vi "GotoWaypoint.vi"(7 "InhibitIn":bool, 8 "CurrentSteerAngle":dbl, 9 "WhatAroundMe? Clean":cluster{"T":dbl, "Range":dbl, "Bearing":dbl}[](array[cluster]), 10 "WhereAmI? Clean":T3, 11 "MDF In":T2(array[cluster])) -> (0 "BehCom":T1(ring), 1 "MDF Out":T2(array[cluster]), 2 "ActCommand":dbl[](array[numeric]), 4 "InhibitOut":bool, 5 "Vel":dbl, 6 "SteerAngle":dbl)   [LabVIEW 2012]
doc: "This subVI contains the Forebrain Goto Waypoint behaviors. Its inputs are the outputs of thewhat and where SENSE processes, theMission efinition Filet, a suppression value from another co-brahvior and an inhibit signal to turn the behavior off. The outputs are a 90 element steering array and a suppression value to diminish the output of co-behaviors.\n\nIt is designed to work with a 90 element behavior arbiter."
uses:
  <vilib>/Analysis/1siggen.llb/Ramp Pattern by Samples.vi
  <vilib>/gmath/statdist.llb/Normal PDF.vi
  <vilib>/gmath/NI_Gmath.lvlib
  <vilib>/Analysis/NI_AALBase.lvlib
panel:
  out "loop index":i32
  in  "HowAmI? Clean":cluster{"T":dbl, "Battery":dbl, "Temp":dbl}
  # "This VI contains the go to waypoint behavior  at the Forebrain level"
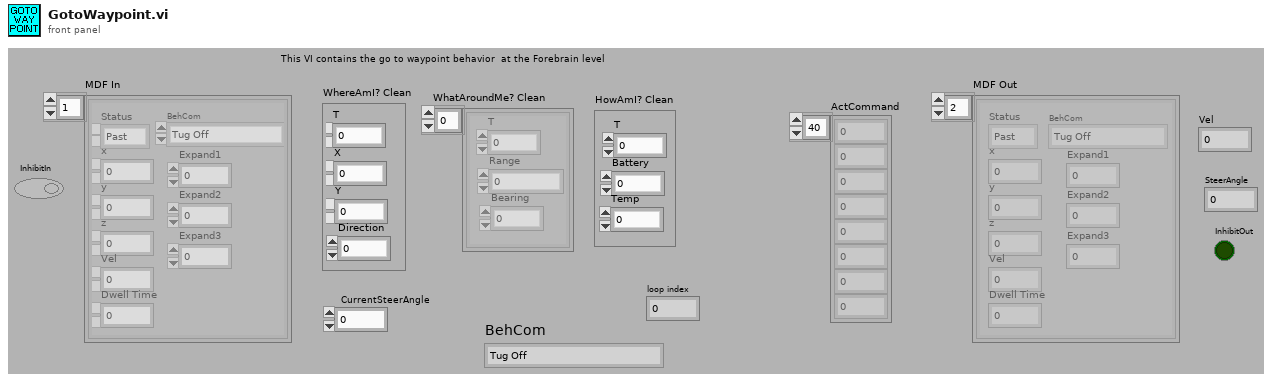
[diagram p1: front panel]
types:
  T1 = enum16{"Tug Off", "Manual Mode", "Goto WayPoint", "Back Up", "Circle", "Left Wall Follow", "Right Wall Follow", "Hunt"}
  T2 = cluster{"Status":enum16{"Past", "Current", "Future"}, "x":dbl, "y":dbl, "z":dbl, "Vel":dbl, "Dwell Time":dbl, "BehCom":enum16{"Tug Off", "Manual Mode", "Goto WayPoint", "Back Up", "Circle", "Left Wall Follow", "Right Wall Follow", "Hunt"}, "Expand1":dbl, "Expand2":dbl, "Expand3":dbl}[]
  T3 = cluster{"T":dbl, "X":dbl, "Y":dbl, "Direction":dbl}
  T4 = cluster{"Status":enum16{"Past", "Current", "Future"}, "x":dbl, "y":dbl, "z":dbl, "Vel":dbl, "Dwell Time":dbl, "BehCom":enum16{"Tug Off", "Manual Mode", "Goto WayPoint", "Back Up", "Circle", "Left Wall Follow", "Right Wall Follow", "Hunt"}, "Expand1":dbl, "Expand2":dbl, "Expand3":dbl}
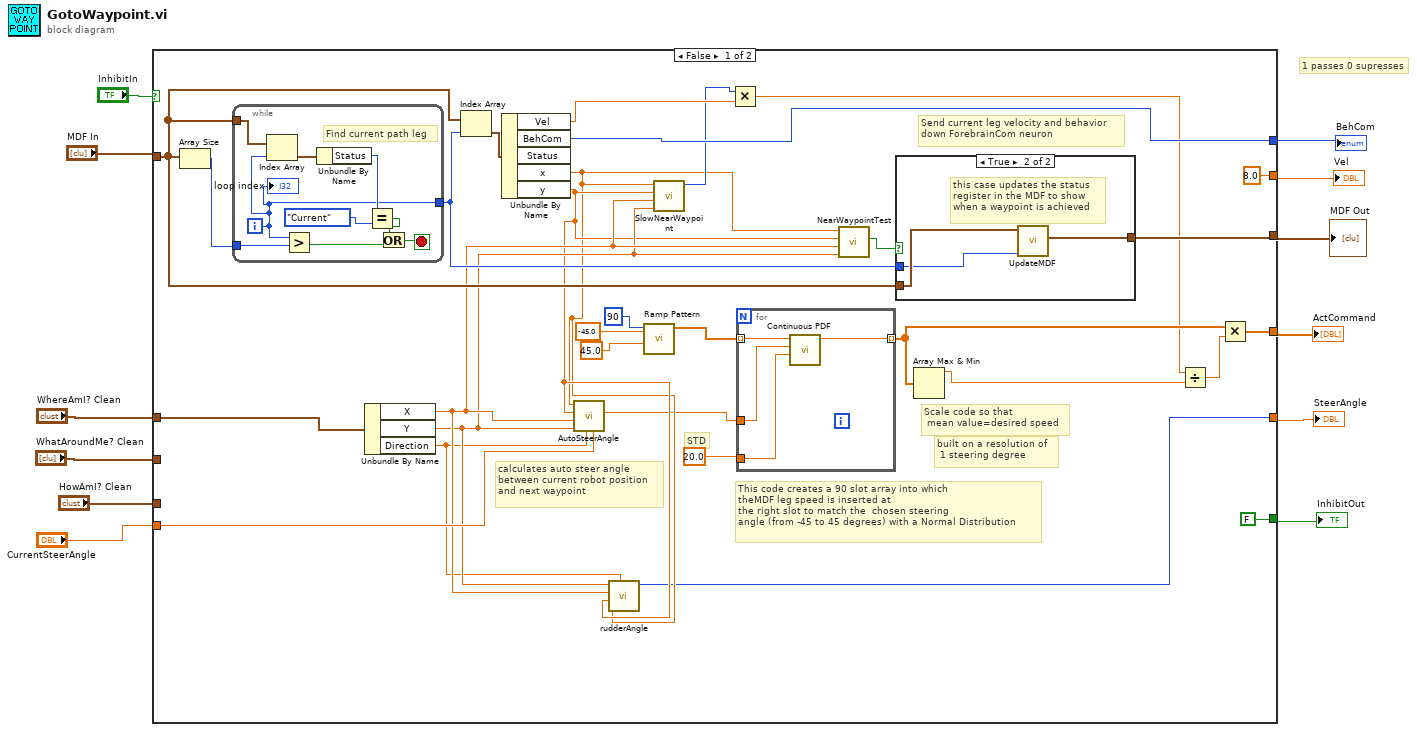
[diagram p0: block diagram]
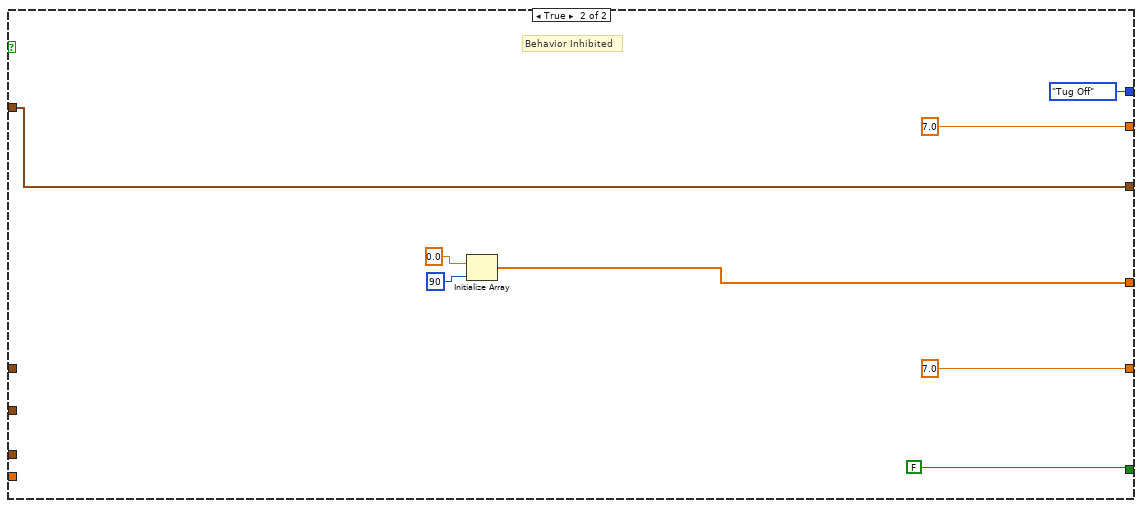
[diagram p3: hidden frame]
diagram:
  # "1 passes 0 supresses"
  n1 = case shown="False" "InhibitIn" {
    tunnel: "WhatAroundMe? Clean" -> [_ _]
    tunnel: "WhereAmI? Clean" -> [w40 _]
    tunnel: "HowAmI? Clean" -> [_ _]
    tunnel: [w30 w66] -> w7
    tunnel: [FALSE ("InhibitOut") FALSE ("InhibitOut")] -> w8
    tunnel: "MDF In" -> [w28 w63]
    tunnel: [w27 w63] -> w5
    tunnel: [8.0 ("Vel") 7.0 ("Vel")] -> w4
    tunnel: [w14 7.0 ("SteerAngle")] -> w3
    tunnel: "CurrentSteerAngle" -> [w25 _]
    tunnel: [w24 T1."Tug Off" ("BehCom")] -> w1
    frame False {
      # "Send current leg velocity and behavior\ndown ForebrainCom neuron"
      # "calculates auto steer angle\nbetween current robot position\nand next waypoint"
      # "built on a resolution of\n 1 steering degree"
      # "Scale code so that\n mean value=desired speed"
      # "STD"
      # "This code creates a 90 slot array into which\ntheMDF leg speed is inserted at\nthe right slot to match the  chosen steering\nangle (from -45 to 45 degrees) with a Normal Distribution"
      n2 = Array Size(array=w28) -> (size(s)=w41:i32)
      n3 = while {
        tunnel: w41 -> [w59]
        tunnel: w28 -> [w56]
        tunnel: [w51] -> w26
        i -> [w51]
        stop <- w58 stop-if-true
        # "Find current path leg"
        n4 = Index Array "Index Array"(array=w56, index=w51) -> (element=w53:T4)
        n5 = Greater?(x=w51, y=w59) -> (0:w57:bool)
        n6 = Unbundle By Name(w53) -> ("Status"=w54:enum16{"Past", "Current", "Future"})
        n7 = Equal?(x=w54, y=enum16{"Past", "Current", "Future"}."Current") -> (x = y?=w55:bool)
        n8 = Or(x=w55, y=w57) -> (x .or. y?=w58:bool)
        "loop index" <- w51
      }
      n9 = Unbundle By Name(w40) -> ("X"=w20:dbl, "Y"=w19:dbl, "Direction"=w18:dbl)
      n10 = Index Array "Index Array"(array=w28, index=w26) -> (element=w39:T4)
      n11 = Unbundle By Name(w39) -> ("Vel"=w23:dbl, "BehCom"=w24:T1, "x"=w16:dbl, "y"=w17:dbl)  [unwired: 1 out]
      n12 = call "AutoSteerAngle.vi"("CurrentSteerAngle"=w25, "CurrentDirection"=w18, "Ycurrent"=w19, "Xcurrent"=w20, "Ywaypoint"=w17, "Xwaypoint"=w16) -> ("NewSteerAngle"=w15:dbl)  [unwired: 5 in]
      n13 = call "rudderAngle.vi"("BoatHeading"=w18, "YGoal"=w16, "XGoal"=w17, "Yboat"=w20, "Xboat"=w19) -> ("RudderAngle"=w14:i16)  [unwired: 1 in, 2 out]
      n14 = call-poly <vilib>:"Ramp Pattern.vi"("start"=45.0, "end"=-45.0 ("end (Normal)"), "samples"=90) -> ("Ramp Pattern"=w33:dbl[])  [unwired: 7 in, 1 out]
      n15 = call "SlowNearWaypoint.vi"("Yrobot"=w19, "Xrobot"=w20, "Ywaypoint"=w17, "Xwaypoiny"=w16) -> ("SpeedDecrease"=w21:i32)  [unwired: 7 in]
      n16 = Multiply(x=w21, y=w23) -> (x*y=w22:dbl)
      n17 = for {
        tunnel: w33 -> [w50] mode=indexing
        tunnel: 20.0 ("std (Normal)") -> [w49]
        tunnel: [w48] -> w37 mode=indexing
        tunnel: w15 -> [w47]
        n18 = call-poly <vilib>:"Continuous PDF.vi"("std"=w49, "mean"=w47, "x"=w50) -> ("pdf(x)"=w48:dbl)  [unwired: 7 in, 1 out]
      }
      n19 = call "NearWaypointTest.vi"("Yrobot"=w19, "Xrobot"=w20, "Ywaypoint"=w17, "Xwaypoiny"=w16) -> ("AtWaypoint"=w29:bool)  [unwired: 7 in]
      n20 = case shown="True" w29 {
        tunnel: w28 -> [w43 w46]
        tunnel: [w43 w44] -> w27
        tunnel: w26 -> [_ w45]
        frame False {
          # "robot not near waypoint\npass MDF through unaltered"
        }
        frame True {
          # "this case updates the status\nregister in the MDF to show \nwhen a waypoint is achieved"
          n21 = call "UpdateMDF.vi"("Index"=w45, "MDF_In"=w46) -> ("MDF_Out"=w44:T2)  [unwired: 9 in]
        }
      }
      n22 = Array Max & Min(array=w37) -> (max value=w35:dbl)  [unwired: 3 out]
      n23 = Divide(x=w22, y=w35) -> (x/y=w36:dbl)
      n24 = Multiply(x=w37, y=w36) -> (x*y=w30:dbl[])
    }
    frame True {
      # "Behavior Inhibited"
      n25 = Initialize Array "Initialize Array"(0.0 ("element"), 90 ("dimension size")) -> (w66:dbl[])
    }
  }
  "ActCommand" <- w7
  "InhibitOut" <- w8
  "MDF Out" <- w5
  "Vel" <- w4
  "SteerAngle" <- w3
  "BehCom" <- w1
